vi "initNewMessage.vi"(7 "path in":path=path "C:/dev/Hexagon-VTD-Custom-Device/Libraries/VC.dll", 8 "error in (no error)":errorcluster, 9 "simFrame":u32, 10 "simTime":dbl, 11 "builderHandle in":u64) -> (0 "error out":errorcluster, 3 "builderHandle out":u64)   [LabVIEW 2023, in "RDB.lvlib"]
uses:
  RDB.lvlib
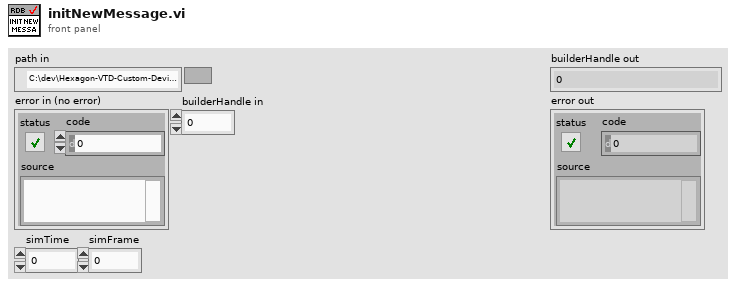
[diagram p1: front panel]
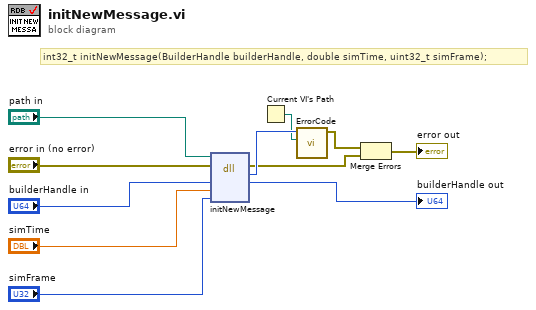
[diagram p0: block diagram]
diagram:
  # "int32_t initNewMessage(BuilderHandle builderHandle, double simTime, uint32_t simFrame);"
  n1 = dll-call lib="C:/dev/Hexagon-VTD-Custom-Device/Libraries/libVC.dll" fn="initNewMessage"(path in="path in", error in="error in (no error)", "builderHandle"="builderHandle in", "simTime"="simTime", "simFrame"="simFrame") -> (error out=w6:errorcluster, "return type"=w8:i32, "builderHandle"=→"builderHandle out":u64)  [unwired: 3 in, 1 out]
  n2 = Current VI's Path() -> (path=w3:path)
  n3 = call "ErrorCode.vi"("parent VI path"=w3, "return type"=w8) -> ("error out"=w7:errorcluster)  [unwired: 9 in]
  n4 = Merge Errors(w7, w6) -> (→"error out":errorcluster)
